vi "ReferencedVariables_ReadWriteReferencedVariable_6x8x6_Singleton.vi"(1 "ReplaceWithtypeDef":dbl, 5 "error in (no error)":errorcluster) -> (19 "error out":errorcluster)   [LabVIEW 2010]
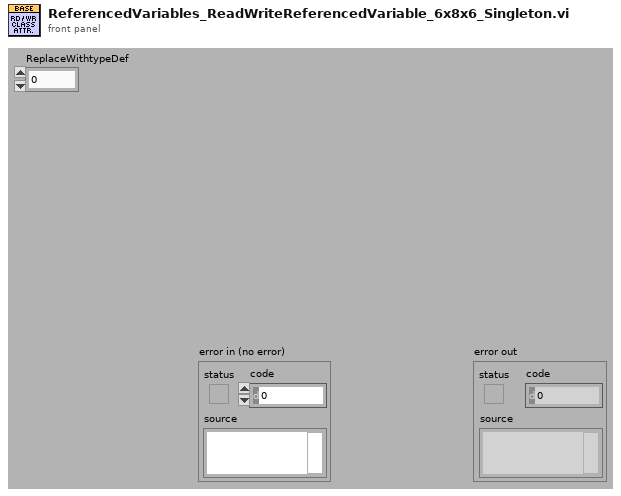
[diagram p1: front panel]
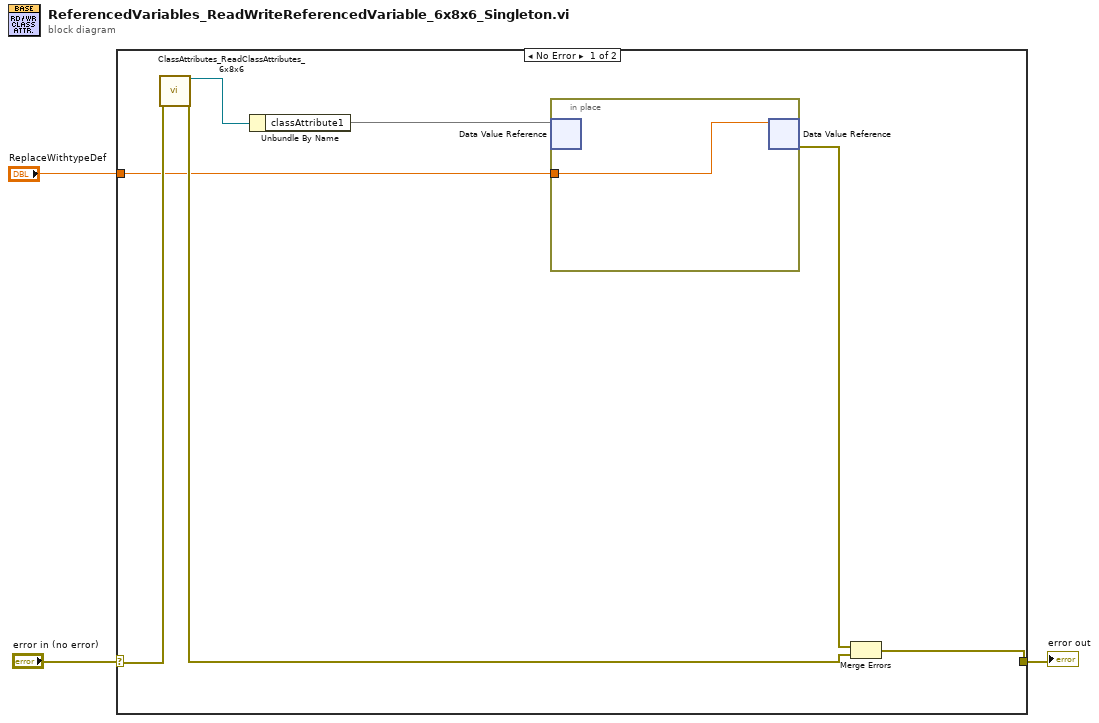
[diagram p0: block diagram]
diagram:
  n1 = case shown="No Error" "error in (no error)" {
    selector: "error in (no error)" -> [w8 w12]
    tunnel: [w9 w12] -> w2
    tunnel: "ReplaceWithtypeDef" -> [w4 _]
    frame No Error {
      n2 = call "ClassAttributes_ReadClassAttributes_6x8x6.vi"("error in (no error)"=w8) -> ("reference out"=w5:refnum<class>, "error out"=w7:errorcluster)  [unwired: 17 in]
      n3 = Unbundle By Name(w5) -> ("classAttribute1"=w6)
      n4 = in-place {
        in-place-border: w4 -> [w11]
        n5 = in-place-dvr #1(w6) -> ()  [unwired: 2 out]
        n6 = in-place-dvr #1(w11) -> (w10:errorcluster)  [unwired: 1 out]
      }
      n7 = Merge Errors(w10, w7) -> (w9:errorcluster)
    }
    frame Error {
    }
  }
  "error out" <- w2
